vi "Set State Description.vi"(8 "error in":errorcluster, 9 "descriptions":string, 10 "state":string, 11 "routing channel in":T1 format="%.0x") -> (0 "error out":errorcluster, 3 "routing channel out":T1=18446744073709551615 format="%.0x")   [LabVIEW 2020, in "Routing and Faulting Scripting.lvlib"]
doc: "Sets the description of the state."
uses:
  Routing and Faulting Scripting.lvlib
  <vilib>/NI VeriStand/Custom Device API/Custom Device Item Ref.ctl
  <vilib>/Utility/error.llb/Error Cluster From Error Code.vi
  <vilib>/NI VeriStand/Custom Device API/Custom Device API.lvlib
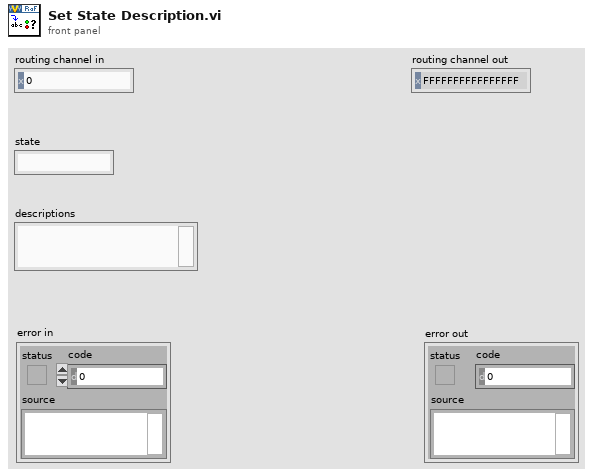
[diagram p1: front panel]
types:
  T1 = typedef "Custom Device API.lvlib/Custom Device Item Ref.ctl" = u64
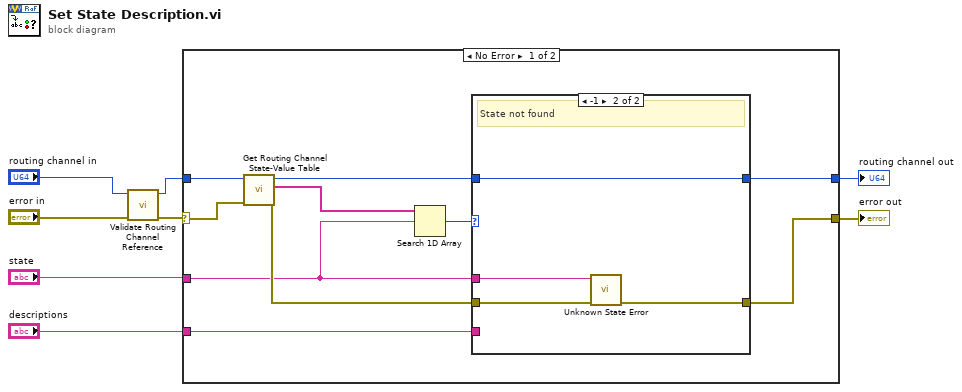
[diagram p0: block diagram]
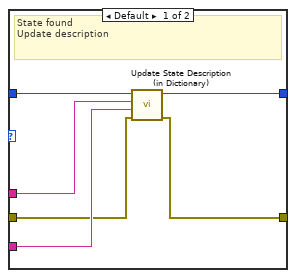
[diagram p2: hidden frame]
diagram:
  n1 = call "Validate Routing Channel Reference.vi"("error in"="error in", "routing channel in"="routing channel in") -> ("error out"=w3:errorcluster, "routing channel out"=w1:T1)  [unwired: 8 in]
  n2 = case shown="No Error" w3 {
    selector: w3 -> [w17 w30]
    tunnel: [w13 w30] -> w5
    tunnel: w1 -> [w18 w29]
    tunnel: [w14 w29] -> w4
    tunnel: "state" -> [w11 _]
    tunnel: "descriptions" -> [w10 _]
    frame No Error {
      n3 = call "Get Routing Channel State-Value Table.vi"("error in"=w17, "routing channel in"=w18) -> ("error out"=w15:errorcluster, "state names"=w12:string[], "routing channel out"=w16:T1)  [unwired: 6 in, 1 out]
      n4 = Search 1D Array(1D array=w12, element=w11) -> (index of element=w9:i32)  [unwired: 1 in]
      n5 = case shown="-1" w9 {
        tunnel: w16 -> [w24 w28]
        tunnel: w15 -> [w20 w27]
        tunnel: [w23 w28] -> w14
        tunnel: [w19 w26] -> w13
        tunnel: w10 -> [w21 _]
        tunnel: w11 -> [w22 w25]
        frame Default {
          # "State found\nUpdate description"
          n6 = call "Update State Description (in Dictionary).vi"("error in"=w20, "description"=w21, "state"=w22, "routing channel in"=w24) -> ("error out"=w19:errorcluster, "routing channel out"=w23:T1)  [unwired: 6 in]
        }
        frame -1 {
          # "State not found"
          n7 = call "Unknown State Error.vi"("error in (no error)"=w27, "state"=w25) -> ("error out"=w26:errorcluster)  [unwired: 9 in]
        }
      }
    }
    frame Error {
    }
  }
  "routing channel out" <- w4
  "error out" <- w5
